vi "settings_filename_to_registry.vi"(10 "Last Used Settings File":string) -> ()   [LabVIEW 2019]
uses:
  <vilib>/registry/registry.llb/Registry RtKey.ctl
  <vilib>/registry/registry.llb/Registry SAM.ctl
  <vilib>/registry/registry.llb/Write Registry Value Simple.vi
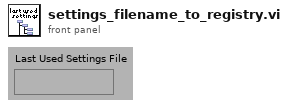
[diagram p1: front panel]
types:
  T1 = typedef "Registry SAM.ctl" = enum32{"KEY_QUERY_VALUE", "KEY_SET_VALUE", "KEY_CREATE_SUB_KEY", "KEY_ENUMERATE_SUB_KEYS", "KEY_NOTIFY", "KEY_CREATE_LINK", "KEY_READ", "KEY_WRITE", "KEY_ALL_ACCESS", "KEY_READ | KEY_WRITE"}
  T2 = typedef "Registry RtKey.ctl" = enum32{"HKEY_CLASSES_ROOT", "HKEY_CURRENT_USER", "HKEY_LOCAL_MACHINE", "HKEY_USERS", "HKEY_PERFORMANCE_DATA", "HKEY_CURRENT_CONFIG", "HKEY_DYN_DATA"}
  T3 = typedef "Registry refnum.ctl" = refnum<k1>
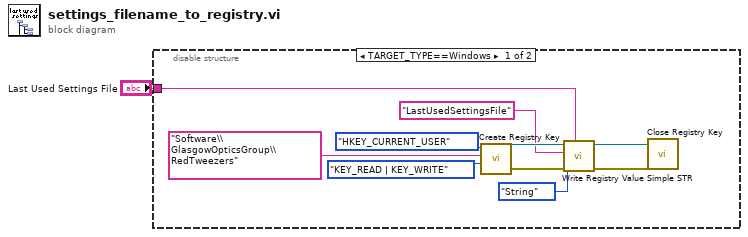
[diagram p0: block diagram]
diagram:
  n1 = disable-structure shown="TARGET_TYPE==Windows" {
    disable-tunnel: "Last Used Settings File" -> [w2 _]
    frame condition #0 (active) {
      n2 = call <vilib>:"Create Registry Key.vi"("security access mask (KEY_READ | KEY_WRITE)"=Registry_SAM."KEY_READ | KEY_WRITE", "subkey"="Software\\GlasgowOpticsGroup\\RedTweezers", "root key (HKEY_LOCAL_MACHINE)"=Registry_RtKey."HKEY_CURRENT_USER") -> ("error out"=w7:errorcluster, "refnum out"=w5:T3)  [unwired: 6 in, 1 out]
      n3 = call-poly <vilib>:"Write Registry Value Simple STR.vi"("String/Binary data"=w2, "error in (no error)"=w7, "simple data type"=enum16{"String", "Binary", "DWORD"}."String", "value"="LastUsedSettingsFile", "refnum"=w5) -> ("error out"=w6:errorcluster, "refnum out"=w4:T3)  [unwired: 3 in]
      n4 = call <vilib>:"Close Registry Key.vi"("error in (no error)"=w6, "refnum"=w4) -> ()  [unwired: 5 in, 1 out]
    }
    frame condition #1 {
    }
  }
